vi "dfd_Set Filter Coef Type.vi"   [LabVIEW 2017, in "NI_DigFilterLicensed.lvlib"]
uses:
  <vilib>/addons/Digital Filter Design/NI_DigFilterLicensed.lvlib
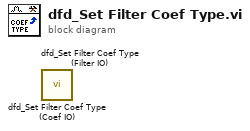
[diagram p0: block diagram]
diagram:
  n1 = call <vilib>:"dfd_Set Filter Coef Type (Coef IO).vi"() -> ()  [unwired: 10 in, 2 out]
  n2 = call <vilib>:"dfd_Set Filter Coef Type (Filter IO).vi"() -> ()  [unwired: 10 in, 2 out]
